vi "GPS Data Loop.vi"() -> ()   [LabVIEW 2011]
uses:
  <instrlib>/NavCom SF-2050/NavCom SF-2050.lvlib
panel:
  in  "error in (no error)":errorcluster
  in  "VISA resource name":refnum<visa-resource-name>
  in  "Debug":bool
  in  "Serial Configuration":cluster{"Baud Rate":u32, "Parity":u16}={"Baud Rate"=115200, "Parity"=0} {"Parity" items=["None", "Odd", "Even", "Mark", "Space"]; "Baud Rate" items=["1200"=1200, "2400"=2400, "4800"=4800, "9600"=9600, "19200"=19200, "38400"=38400, "57600"=57600, "115200"=115200]}
  in  "GPS Data 2":T1 {"Time"."GPS Time of Week" format="%.3f"; "Velocity, Correction & SET"."Extended Navigation Mode" items=["Non Differential"=0, "Code (RTCM Type 1 & 9)"=1, "Code, Single Frequency (WAAS)"=2, "Code, Dual Frequency (WAAS)"=3, "Code, Single Frequency (WCT)"=4, "Code/RCP, Dual Frequency (WCT)"=5, "Code, Single Frequency (RTG)"=6, "Code (RTCM Type 1 & 9) Dual Frequency"=10, "Code/RCP, Dual Frequency (RTG)"=11, "Code, Single Frequency (NCT-RTK)"=12, "Code, Single Frequency (RTCM 18 & 19)"=13, "Code, Single Frequency (RTCM 21 & 22)"=14, "Code, Single Frequency (CMR)"=15, "Code, Dual Frequency (NCT-RTK)"=16, "Code, Dual Frequency (RTCM 18 & 19)"=17, "Code, Dual Frequency (RTCM 20 & 21)"=18, "Code, Dual Frequency (CMR)"=19, "RTK (NCT-RTK)"=20, "RTK (RTCM 18 & 19)"=21, "RTK (RTCM 20 & 21)"=22, "RTK (CMR)"=23, "Code, Single Frequency with SET (RTG)"=24, "Code/RCP, Dual Frequency with SET (RTG)"=25, "RTK Extend"=26]}
  out "GPS Data":T1 {"Time"."GPS Time of Week" format="%.3f"; "Velocity, Correction & SET"."Extended Navigation Mode" items=["Non Differential"=0, "Code (RTCM Type 1 & 9)"=1, "Code, Single Frequency (WAAS)"=2, "Code, Dual Frequency (WAAS)"=3, "Code, Single Frequency (WCT)"=4, "Code/RCP, Dual Frequency (WCT)"=5, "Code, Single Frequency (RTG)"=6, "Code (RTCM Type 1 & 9) Dual Frequency"=10, "Code/RCP, Dual Frequency (RTG)"=11, "Code, Single Frequency (NCT-RTK)"=12, "Code, Single Frequency (RTCM 18 & 19)"=13, "Code, Single Frequency (RTCM 21 & 22)"=14, "Code, Single Frequency (CMR)"=15, "Code, Dual Frequency (NCT-RTK)"=16, "Code, Dual Frequency (RTCM 18 & 19)"=17, "Code, Dual Frequency (RTCM 20 & 21)"=18, "Code, Dual Frequency (CMR)"=19, "RTK (NCT-RTK)"=20, "RTK (RTCM 18 & 19)"=21, "RTK (RTCM 20 & 21)"=22, "RTK (CMR)"=23, "Code, Single Frequency with SET (RTG)"=24, "Code/RCP, Dual Frequency with SET (RTG)"=25, "RTK Extend"=26]; "Altitude" format="%#_18g"; "Longitude" format="%#_18g"; "Latitude" format="%#_18g"}
  out "error out":errorcluster
  in  "stop?":bool
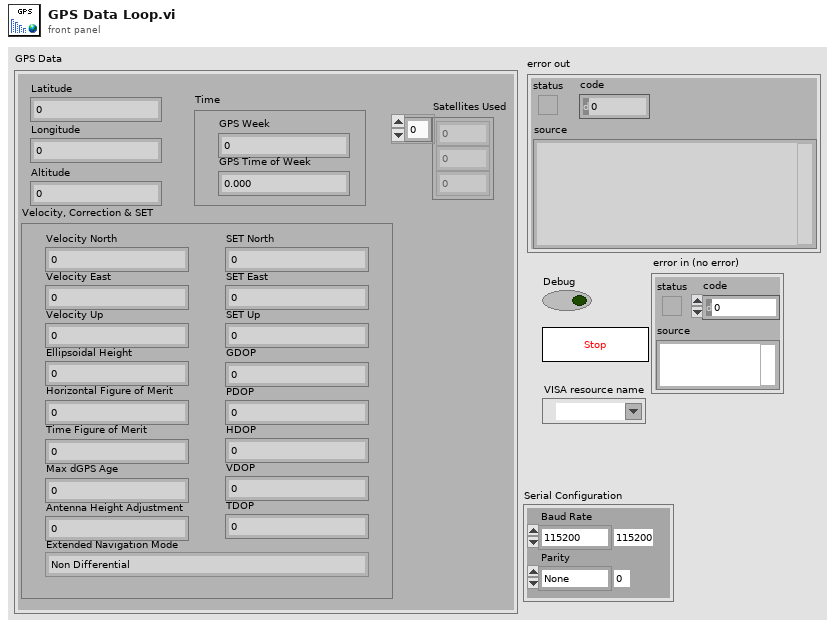
[diagram p1: front panel]
types:
  T1 = cluster{"Latitude":dbl, "Longitude":dbl, "Altitude":dbl, "Velocity, Correction & SET":cluster{"Velocity North":dbl, "Velocity East":dbl, "Velocity Up":dbl, "Ellipsoidal Height":dbl, "GDOP":sgl, "PDOP":sgl, "HDOP":sgl, "VDOP":sgl, "TDOP":sgl, "Horizontal Figure of Merit":u8, "Time Figure of Merit":u8, "Max dGPS Age":sgl, "Extended Navigation Mode":u8, "Antenna Height Adjustment ":dbl, "SET North":i32, "SET East":i32, "SET Up":i32}, "Time":cluster{"GPS Week":u16, "GPS Time of Week":sgl}, "Satellites Used":i32[]}
  T2 = cluster{"Velocity North":dbl, "Velocity East":dbl, "Velocity Up":dbl, "Ellipsoidal Height":dbl, "GDOP":sgl, "PDOP":sgl, "HDOP":sgl, "VDOP":sgl, "TDOP":sgl, "Horizontal Figure of Merit":u8, "Time Figure of Merit":u8, "Max dGPS Age":sgl, "Extended Navigation Mode":u8, "Antenna Height Adjustment ":dbl, "SET North":i32, "SET East":i32, "SET Up":i32}
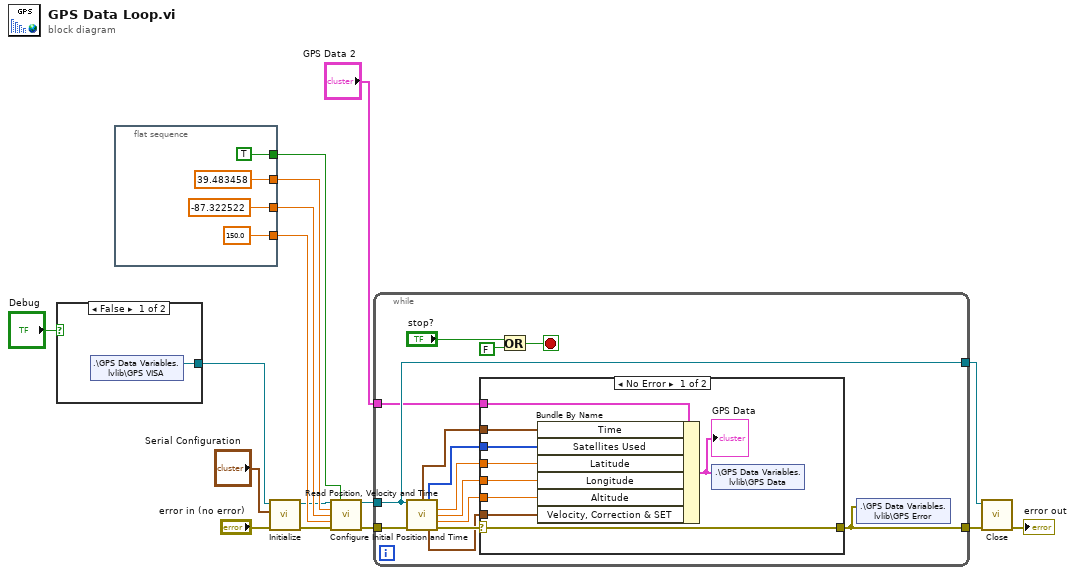
[diagram p0: block diagram]
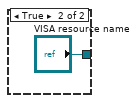
[diagram p3: hidden frame]
diagram:
  n1 = case shown="False" "Debug" {
    tunnel: [w17 "VISA resource name"] -> w4
    frame False {
      n2 = shared-variable ".\\GPS Data Variables.lvlib\\GPS VISA"() -> (w17:refnum<visa-resource-name>)  [unwired: 1 in, 1 out]
    }
    frame True {
    }
  }
  n3 = flat-sequence {
    tunnel: [39.483458 ("Initial Latitude (0°)")] -> w11
    tunnel: [-87.322522 ("Initial Latitude (0°)")] -> w10
    tunnel: [sgl 150.0 ("Initial Ellipsoidal Height (0 meters)")] -> w9
    tunnel: [TRUE ("Enable Set Initial Position")] -> w8
    frame #0 {
    }
  }
  n4 = call <instrlib>:"Initialize.vi"("error in (no error)"="error in (no error)", "Serial Configuration"="Serial Configuration", "VISA resource name"=w4) -> ("error out"=w2:errorcluster, "VISA resource name out"=w3:refnum<visa-resource-name>)  [unwired: 7 in]
  n5 = call <instrlib>:"Configure Initial Position and Time.vi"("VISA resource name"=w3, "Enable Set Initial Position"=w8, "Initial Latitude (0°)"=w11, "Initial Longitude (0°)"=w10, "Initial Ellipsoidal Height (0 meters)"=w9, "error in (no error)"=w2) -> ("VISA resource name out"=w7:refnum<visa-resource-name>, "error out"=w6:errorcluster)  [unwired: 8 in]
  n6 = while {
    tunnel: w7 -> [w34]
    tunnel: w6 -> [w35]
    tunnel: [w34] -> w16
    tunnel: [w23] -> w15
    tunnel: "GPS Data 2" -> [w31]
    stop <- w32 stop-if-true
    n7 = call <instrlib>:"Read Position, Velocity and Time.vi"("VISA resource name"=w34, "error in (no error)"=w35) -> ("Time"=w25:cluster{"GPS Week":u16, "GPS Time of Week":sgl}, "Satellites Used"=w26:i32[], "Latitude"=w30:dbl, "Longitude"=w29:dbl, "Altitude"=w28:dbl, "Velocity, Correction & SET"=w27:T2, "error out"=w33:errorcluster)  [unwired: 6 in, 1 out]
    n8 = case shown="No Error" w33 {
      selector: w33 -> [w45 w46]
      tunnel: [w45 w46] -> w23
      tunnel: w31 -> [w44 _]
      tunnel: w30 -> [w43 _]
      tunnel: w29 -> [w42 _]
      tunnel: w28 -> [w41 _]
      tunnel: w27 -> [w40 _]
      tunnel: w26 -> [w39 _]
      tunnel: w25 -> [w38 _]
      frame No Error {
        n9 = Bundle By Name(cluster=w44, "Time"=w38, "Satellites Used"=w39, "Latitude"=w43, "Longitude"=w42, "Altitude"=w41, "Velocity, Correction & SET"=w40) -> (w37:T1)
        "GPS Data" <- w37
        n10 = shared-variable ".\\GPS Data Variables.lvlib\\GPS Data"(w37) -> ()  [unwired: 1 in, 1 out]
      }
      frame Error {
      }
    }
    n11 = Or(x="stop?", y=FALSE) -> (x .or. y?=w32:bool)
    n12 = shared-variable ".\\GPS Data Variables.lvlib\\GPS Error"(w23) -> ()  [unwired: 1 in, 1 out]
  }
  n13 = call <instrlib>:"Close.vi"("error in (no error)"=w15, "VISA resource name"=w16) -> ("error out"=→"error out":errorcluster)  [unwired: 9 in]
